vi "CRC_Attach.vi"(2 "error in (no error)":errorcluster caption="错误输入（无错误）", 3 "info_data":dbl[](array[numeric]), 4 "path":path) -> (0 "error out":errorcluster caption="错误输出", 1 "crc_data":dbl[](array[numeric]))   [LabVIEW 2015]
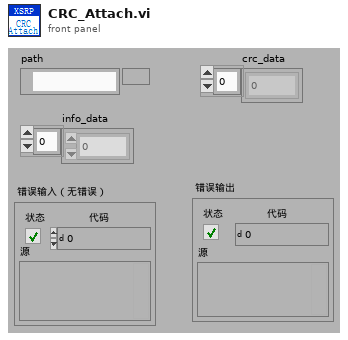
[diagram p1: front panel]
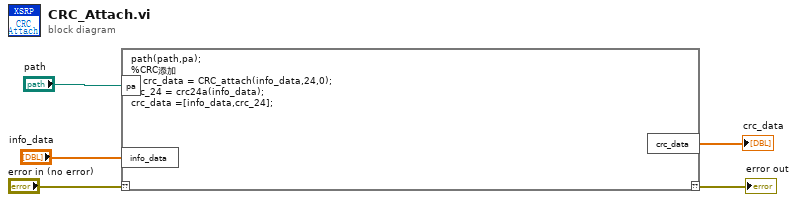
[diagram p0: block diagram]
diagram:
  n1 = script code="path(path,pa);\n%CRC添加\n% crc_data = CRC_attach(info_data,24,0);\ncrc_24 = crc24a(info_data);\ncrc_data =[info_data,crc_24];"("??"="error in (no error)", "pa"="path", "info_data"="info_data") -> ("??"=→"error out":errorcluster, "crc_data"=→"crc_data":dbl[])
